vi "KE6221 -- Get Sine Wave Params.vi"(0 "Resource In":refnum<visa-resource-name>, 1 "Check For SCPI Errors? (T)":bool=TRUE, 11 "error in (no error)":errorcluster) -> (4 "Resource Out (dupl)":refnum<visa-resource-name>, 8 "Sine Wave Params":T1={"Frequency (Hz)"=1000.0, "Amplitude (A)"=0.001, "Offset (A)"=0.0, "Ranging Mode"=enum."Best", "Fixed Range"=enum."2mA", "Playback Mode"=enum."Time", "Time (s)"=1.0, "Num Cycles"=1.0, "Phase\nMarker?"=FALSE, "Phase Marker (deg)"=180.0, "Trig Link Line"=enum."1"} {"Offset (A)" min=-0.105 max=0.105 format="%.4p"; "Num Cycles" min=0.001 max=99999999900.0 format="%.3p"; "Time (s)" min=1e-07 max=999999.999 format="%.3p"; "Phase Marker (deg)" min=0.0 max=360.0 format="%.3f"; "Amplitude (A)" min=2e-12 max=0.105 format="%.3p"; "Frequency (Hz)" min=0.001 max=100000.0 format="%.3p"}, 15 "error out":errorcluster)   [LabVIEW 2019, in "Keithley 622x.lvlib"]
doc: "Returns the parameters for a sine wave. Note that this VI can only be used with the 6221, since the 6220 doesn't support this feature."
uses:
  Keithley 622x.lvlib
  Typedefs/KE6221 -- Wave Sine Wave Params.ctl
  Low Level/Typedefs/KE6221 -- Wave Frequency.ctl
  Low Level/Typedefs/KE6221 -- Wave Amplitude.ctl
  Source/Typedefs/KE622x -- Current Level.ctl
  Low Level/Typedefs/KE6221 -- Wave Ranging Mode.ctl
  Source/Typedefs/KE622x -- Current Ranges.ctl
  Low Level/Typedefs/KE6221 -- Wave Playback Mode.ctl
  Low Level/Typedefs/KE6221 -- Wave Playback Time.ctl
  Low Level/Typedefs/KE6221 -- Wave Playback Num Cycles.ctl
  Low Level/Typedefs/KE6221 -- Wave Phase Marker.ctl
  Trigger/Low Level/Typedefs/KE622x -- Trig Link Line.ctl
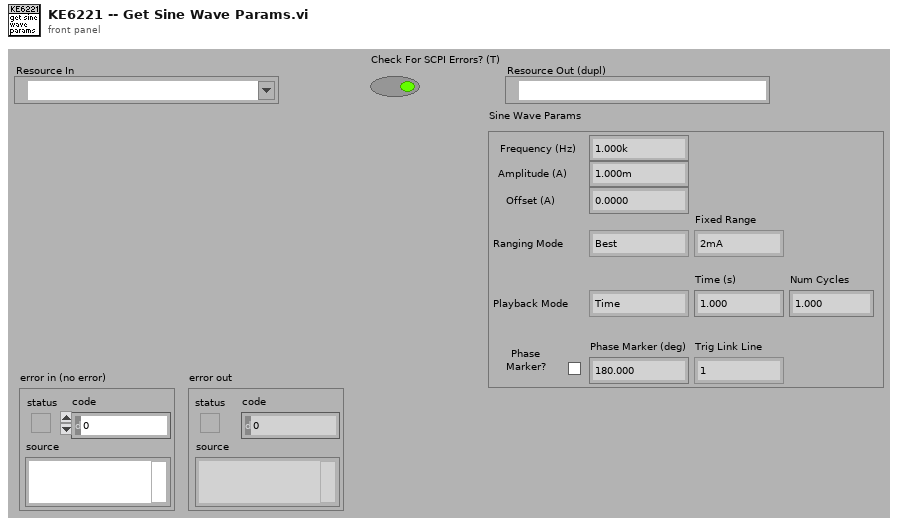
[diagram p1: front panel]
types:
  T1 = typedef "Keithley 622x.lvlib/KE6221 -- Wave Sine Wave Params.ctl" = cluster{"Frequency (Hz)":T2, "Amplitude (A)":T3, "Offset (A)":T4, "Ranging Mode":T5, "Fixed Range":T6, "Playback Mode":T7, "Time (s)":T8, "Num Cycles":T9, "Phase\nMarker?":bool, "Phase Marker (deg)":T10, "Trig Link Line":T11}
  T2 = typedef "Keithley 622x.lvlib/KE6221 -- Wave Frequency.ctl" = dbl
  T3 = typedef "Keithley 622x.lvlib/KE6221 -- Wave Amplitude.ctl" = dbl
  T4 = typedef "Keithley 622x.lvlib/KE622x -- Current Level.ctl" = dbl
  T5 = typedef "Keithley 622x.lvlib/KE6221 -- Wave Ranging Mode.ctl" = enum16{"Best", "Fixed"}
  T6 = typedef "Keithley 622x.lvlib/KE622x -- Current Ranges.ctl" = enum16{"2nA", "20nA", "200nA", "2uA", "20uA", "200uA", "2mA", "20mA", "100mA"}
  T7 = typedef "Keithley 622x.lvlib/KE6221 -- Wave Playback Mode.ctl" = enum16{"Time", "Num Cycles"}
  T8 = typedef "Keithley 622x.lvlib/KE6221 -- Wave Playback Time.ctl" = dbl
  T9 = typedef "Keithley 622x.lvlib/KE6221 -- Wave Playback Num Cycles.ctl" = dbl
  T10 = typedef "Keithley 622x.lvlib/KE6221 -- Wave Phase Marker.ctl" = dbl
  T11 = typedef "Keithley 622x.lvlib/KE622x -- Trig Link Line.ctl" = enum16{"1", "2", "3", "4", "5", "6"}
  T12 = typedef "Keithley 622x.lvlib/KE622x -- Current Range.ctl" = cluster{"Auto Range?":bool, "Man / Selected\nRange":T6}
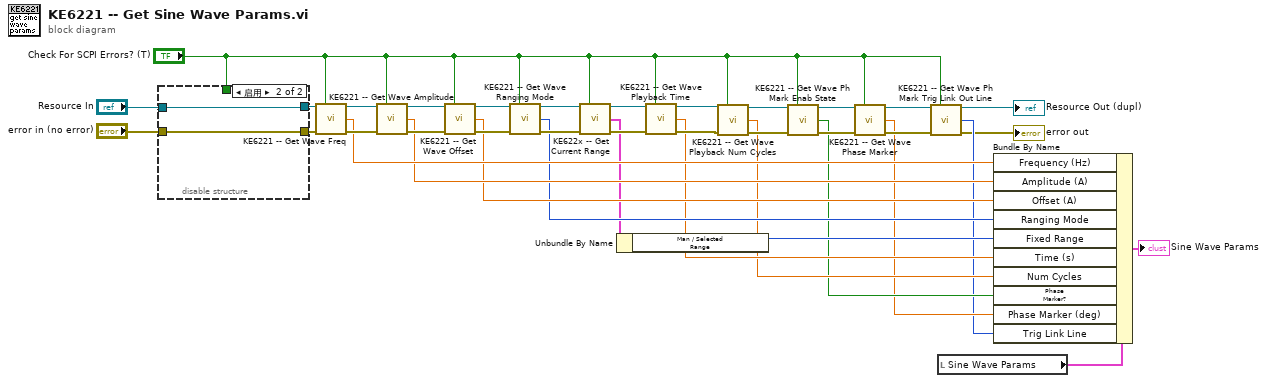
[diagram p0: block diagram]
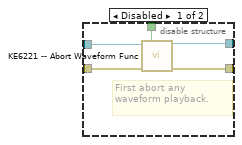
[diagram p2: hidden frame]
diagram:
  n1 = disable-structure shown="启用" {
    disable-tunnel: [w43 w45] -> w5
    disable-tunnel: [w42 w44] -> w4
    disable-tunnel: "Resource In" -> [w41 w45]
    disable-tunnel: "error in (no error)" -> [w40 w44]
    disable-tunnel: "Check For SCPI Errors? (T)" -> [w39 _]
    frame Disabled {
      # "First abort any\nwaveform playback."
      n2 = call "KE6221 -- Abort Waveform Func.vi"("Resource In"=w41, "Check For SCPI Errors? (T)"=w39, "error in (no error)"=w40) -> ("Resource Out (dupl)"=w43:refnum<visa-resource-name>, "error out"=w42:errorcluster)  [unwired: 11 in]
    }
    frame Enabled {
    }
  }
  n3 = call "KE6221 -- Get Wave Freq.vi"("Resource In"=w5, "Check For SCPI Errors? (T)"="Check For SCPI Errors? (T)", "error in (no error)"=w4) -> ("Resource Out (dupl)"=w38:refnum<visa-resource-name>, "KE6221 Wave Freq (Hz)"=w19:T2, "error out"=w37:errorcluster)  [unwired: 10 in]
  n4 = call "KE6221 -- Get Wave Amplitude.vi"("Resource In"=w38, "Check For SCPI Errors? (T)"="Check For SCPI Errors? (T)", "error in (no error)"=w37) -> ("Resource Out (dupl)"=w34:refnum<visa-resource-name>, "Wave Amplitude"=w18:T3, "error out"=w33:errorcluster)  [unwired: 10 in]
  n5 = call "KE6221 -- Get Wave Offset.vi"("Resource In"=w34, "Check For SCPI Errors? (T)"="Check For SCPI Errors? (T)", "error in (no error)"=w33) -> ("Resource Out (dupl)"=w32:refnum<visa-resource-name>, "Wave Offset (A)"=w17:T4, "error out"=w31:errorcluster)  [unwired: 10 in]
  n6 = call "KE6221 -- Get Wave Ranging Mode.vi"("Resource In"=w32, "Check For SCPI Errors? (T)"="Check For SCPI Errors? (T)", "error in (no error)"=w31) -> ("Resource Out (dupl)"=w36:refnum<visa-resource-name>, "Ranging Mode"=w16:T5, "error out"=w35:errorcluster)  [unwired: 10 in]
  n7 = call "KE622x -- Get Current Range.vi"("Resource In"=w36, "Check For SCPI Errors? (T)"="Check For SCPI Errors? (T)", "error in (no error)"=w35) -> ("Resource Out (dupl)"=w30:refnum<visa-resource-name>, "Current Range"=w15:T12, "error out"=w29:errorcluster)  [unwired: 10 in]
  n8 = Unbundle By Name(w15) -> ("Man / Selected\nRange"=w14:T6)
  n9 = call "KE6221 -- Get Wave Playback Time.vi"("Resource In"=w30, "Check For SCPI Errors? (T)"="Check For SCPI Errors? (T)", "error in (no error)"=w29) -> ("Resource Out (dupl)"=w28:refnum<visa-resource-name>, "Playback Time (s)"=w13:T8, "error out"=w27:errorcluster)  [unwired: 10 in]
  n10 = call "KE6221 -- Get Wave Playback Num Cycles.vi"("Resource In"=w28, "Check For SCPI Errors? (T)"="Check For SCPI Errors? (T)", "error in (no error)"=w27) -> ("Resource Out (dupl)"=w26:refnum<visa-resource-name>, "Num Cycles"=w12:T9, "error out"=w25:errorcluster)  [unwired: 10 in]
  n11 = call "KE6221 -- Get Wave Ph Mark Enab State.vi"("Resource In"=w26, "Check For SCPI Errors? (T)"="Check For SCPI Errors? (T)", "error in (no error)"=w25) -> ("Resource Out (dupl)"=w24:refnum<visa-resource-name>, "Phase Marker Enabled?"=w11:bool, "error out"=w23:errorcluster)  [unwired: 10 in]
  n12 = call "KE6221 -- Get Wave Phase Marker.vi"("Resource In"=w24, "Check For SCPI Errors? (T)"="Check For SCPI Errors? (T)", "error in (no error)"=w23) -> ("Resource Out (dupl)"=w22:refnum<visa-resource-name>, "Phase Marker (deg)"=w10:T10, "error out"=w21:errorcluster)  [unwired: 10 in]
  n13 = call "KE6221 -- Get Wave Ph Mark Trig Link Out Line.vi"("Resource In"=w22, "Check For SCPI Errors? (T)"="Check For SCPI Errors? (T)", "error in (no error)"=w21) -> ("Resource Out (dupl)"=→"Resource Out (dupl)":refnum<visa-resource-name>, "Trig Link Out Line"=w9:T11, "error out"=→"error out":errorcluster)  [unwired: 10 in]
  n14 = local read "Sine Wave Params"() -> (w20:T1)
  n15 = Bundle By Name(cluster=w20, "Frequency (Hz)"=w19, "Amplitude (A)"=w18, "Offset (A)"=w17, "Ranging Mode"=w16, "Fixed Range"=w14, "Time (s)"=w13, "Num Cycles"=w12, "Phase\nMarker?"=w11, "Phase Marker (deg)"=w10, "Trig Link Line"=w9) -> (→"Sine Wave Params":T1)
